vi "String decoding.vi"(9 "Decode Status (F)/ Decode Data (T)":bool, 10 "Decode Stability Sign":bool, 11 "Input string":string) -> (0 "Stability sign":string="-", 1 "Unit":string, 2 "Value":dbl, 3 "Status":string, 5 "ID":string)   [LabVIEW 2017, in "RadWag balances and scales.lvlib"]
doc: "Decodes string read from port, and separates it to parts such ass value, unit, stability sign, command ID and status."
uses:
  <instrlib>/Prev/RadWag Continuous Read Folder/RadWag balances and scales.lvlib
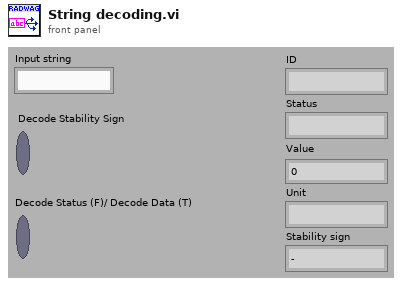
[diagram p1: front panel]
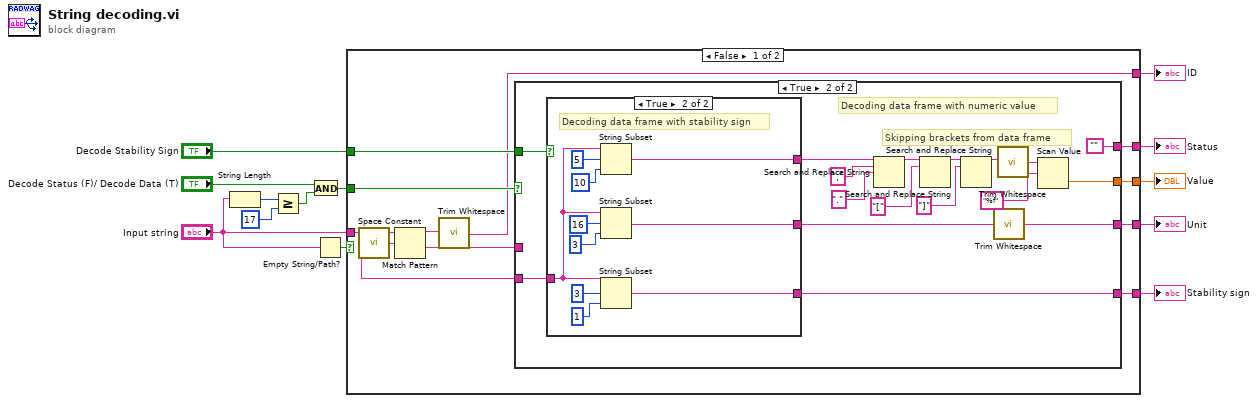
[diagram p0: block diagram]
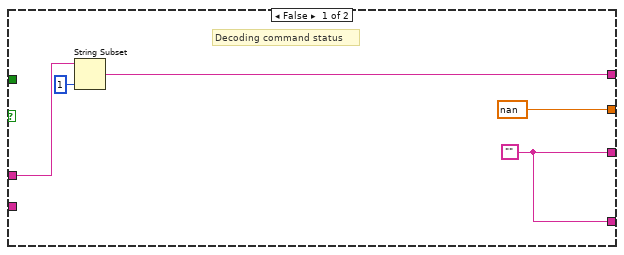
[diagram p2: hidden frame]
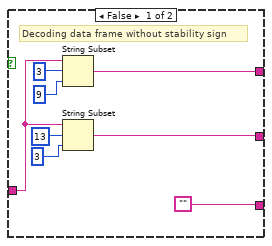
[diagram p3: hidden frame]
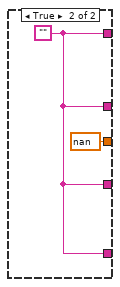
[diagram p4: hidden frame]
diagram:
  n1 = String Length(string="Input string") -> (length=w2:i32)
  n2 = Greater Or Equal?(x=w2, y=17) -> (x >= y?=w3:bool)
  n3 = And(x="Decode Status (F)/ Decode Data (T)", y=w3) -> (x .and. y?=w4:bool)
  n4 = Empty String/Path?(string/path="Input string") -> (empty?=w13:bool)
  n5 = case shown="False" w13 {
    tunnel: "Input string" -> [w22 _]
    tunnel: "Decode Stability Sign" -> [w20 _]
    tunnel: w4 -> [w19 _]
    tunnel: [w18 nan] -> w11
    tunnel: [w17 w66] -> w10
    tunnel: [w16 w66] -> w9
    tunnel: [w15 w66] -> w8
    tunnel: [w14 w66] -> w7
    frame False {
      n6 = call <vilib>:"Space Constant.vi"() -> ("String"=w23:string)
      n7 = Match Pattern(string=w22, regular expression=w23) -> (before substring=w21:string, after substring=w24:string)  [unwired: 1 in, 2 out]
      n8 = call <vilib>:"Trim Whitespace.vi"("string"=w21) -> ("trimmed string"=w14:string)  [unwired: 1 in]
      n9 = case shown="True" w19 {
        tunnel: w24 -> [w28 _]
        tunnel: w22 -> [_ w42]
        tunnel: w20 -> [_ w34]
        tunnel: [nan w33] -> w18
        tunnel: [w25 w32] -> w17
        tunnel: [w25 w31] -> w16
        tunnel: [w27 ""] -> w15
        frame False {
          w25 = ""
          # "Decoding command status"
          n10 = String Subset(string=w28, length (rest)=1 ("length (rest)")) -> (substring=w27:string)  [unwired: 1 in]
        }
        frame True {
          # "Skipping brackets from data frame"
          # "Decoding data frame with numeric value"
          n11 = case shown="True" w34 {
            tunnel: w42 -> [w48 w56]
            tunnel: [w52 w62] -> w45
            tunnel: [w49 w57] -> w41
            tunnel: ["" w55] -> w31
            frame False {
              # "Decoding data frame without stability sign"
              n12 = String Subset(string=w48, offset (0)=3, length (rest)=9 ("length (rest)")) -> (substring=w52:string)
              n13 = String Subset(string=w48, offset (0)=13, length (rest)=3 ("length (rest)")) -> (substring=w49:string)
            }
            frame True {
              # "Decoding data frame with stability sign"
              n14 = String Subset(string=w56, offset (0)=5, length (rest)=10 ("length (rest)")) -> (substring=w62:string)
              n15 = String Subset(string=w56, offset (0)=16, length (rest)=3 ("length (rest)")) -> (substring=w57:string)
              n16 = String Subset(string=w56, offset (0)=3, length (rest)=1 ("length (rest)")) -> (substring=w55:string)
            }
          }
          n17 = Search and Replace String(input string=w45, search string=",", replace string="." ("replace string (\"\")")) -> (result string=w38:string)  [unwired: 5 in, 3 out]
          n18 = Search and Replace String(input string=w38, search string="[") -> (result string=w40:string)  [unwired: 6 in, 3 out]
          n19 = Search and Replace String(input string=w40, search string="]") -> (result string=w39:string)  [unwired: 6 in, 3 out]
          n20 = call <vilib>:"Trim Whitespace.vi"("string"=w41) -> ("trimmed string"=w32:string)  [unwired: 1 in]
          n21 = call <vilib>:"Trim Whitespace.vi"("string"=w39) -> ("trimmed string"=w37:string)  [unwired: 1 in]
          n22 = Scan Value(string=w37, format string="%f") -> (value=w33:dbl)  [unwired: 1 in, 1 out]
        }
      }
    }
    frame True {
      w66 = ""
    }
  }
  "Value" <- w11
  "Unit" <- w10
  "Stability sign" <- w9
  "Status" <- w8
  "ID" <- w7
